vi "Log Data.vi"(8 "error in (no error)":errorcluster, 11 "Sensor & Control in":refnum<class "Sensor.lvclass">) -> (0 "error out":errorcluster, 3 "Sensor & Control out":refnum<class "Sensor.lvclass">)   [LabVIEW 2013, in "Sensor.lvib.lvlib" / "Sensor.lvclass"]
uses:
  Sensor.lvclass
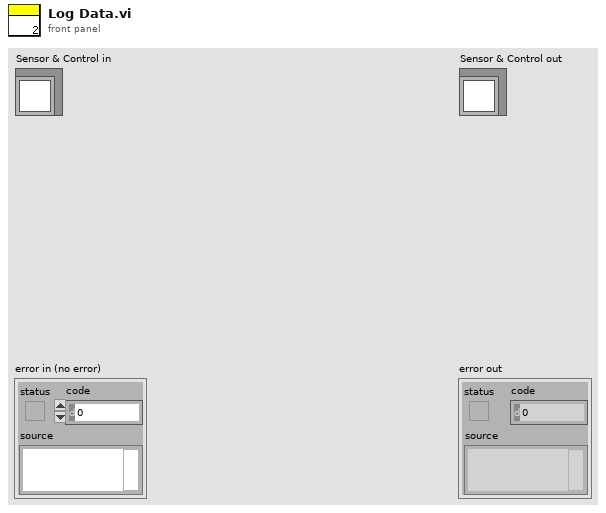
[diagram p1: front panel]
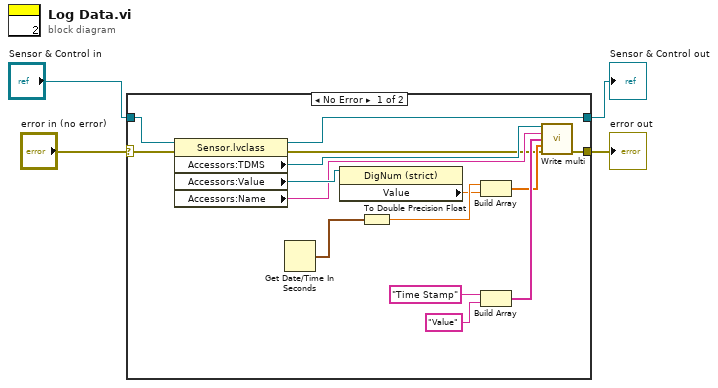
[diagram p0: block diagram]
diagram:
  n1 = case shown="No Error" "error in (no error)" {
    selector: "error in (no error)" -> [w12 w21]
    tunnel: [w11 w21] -> w3
    tunnel: [w5 w20] -> w1
    tunnel: "Sensor & Control in" -> [w18 w20]
    frame No Error {
      n2 = property class="Sensor.lvclass"(reference=w18, error in=w12) -> (reference out=w5:refnum<class "Sensor.lvclass">, error out=w6:errorcluster, "Accessors:TDMS"=w17:refnum<k34>, "Accessors:Value"=w10:refnum<vi>, "Accessors:Name"=w7:string)
      n3 = Get Date/Time In Seconds() -> (seconds since 1Jan1904=w19:timestamp)
      n4 = property class="DigNum (strict)"(reference=w10) -> ("Value"=w9:dbl)  [unwired: 1 in, 2 out]
      n5 = To Double Precision Float(number=w19) -> (double precision float=w13:dbl)
      n6 = Build Array(w13, w9) -> (w8:dbl[])
      n7 = Build Array("Time Stamp" ("Channel"), "Value" ("string")) -> (w14:string[])
      n8 = call "Write multi.vi"("tdms file in"=w17, "group"=w7, "Channel"=w14, "Data"=w8, "error in (no error)"=w6) -> ("error out"=w11:errorcluster)  [unwired: 7 in, 3 out]
    }
    frame Error {
    }
  }
  "error out" <- w3
  "Sensor & Control out" <- w1
